vi "Create System Config Files.vi"(4 "IO's config":string="test setting", 6 "Test Setting":string="test setting", 8 "count":string="Calib", 9 "Settings":string="Settings", 10 "User Data":string="user data", 11 "file path (use dialog)":path=path "C:/Documents and Settings/Owner/Desktop") -> (3 "Path 2":T1)   [LabVIEW 2023]
uses:
  Controls/all path.ctl
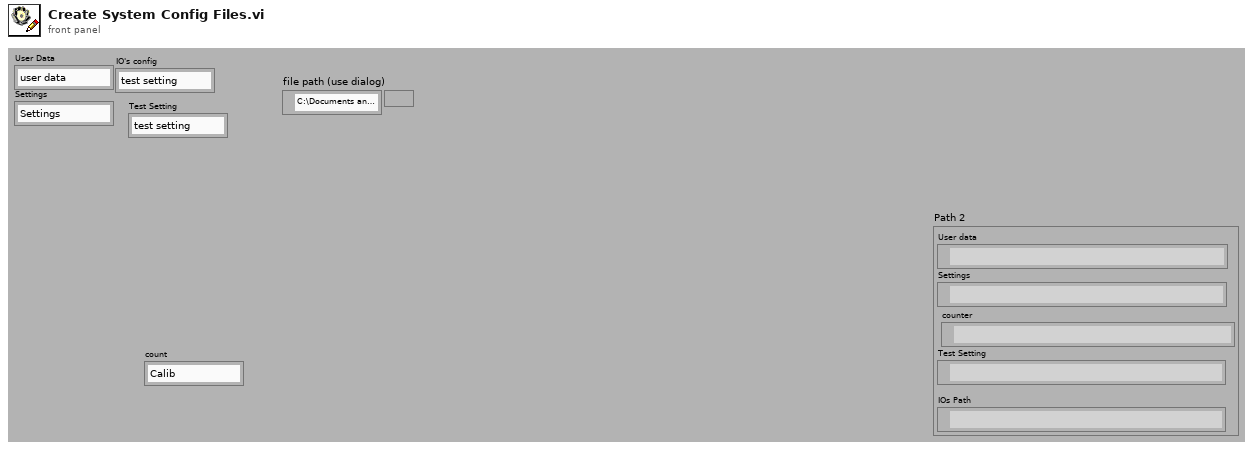
[diagram p1: front panel]
types:
  T1 = typedef "all path.ctl" = cluster{"User data":path, "Settings":path, "counter":path, "Test Setting":path, "IOs Path":path}
  T2 = enum16{"open", "replace", "create", "open or create", "replace or create", "replace or create with confirmation"}
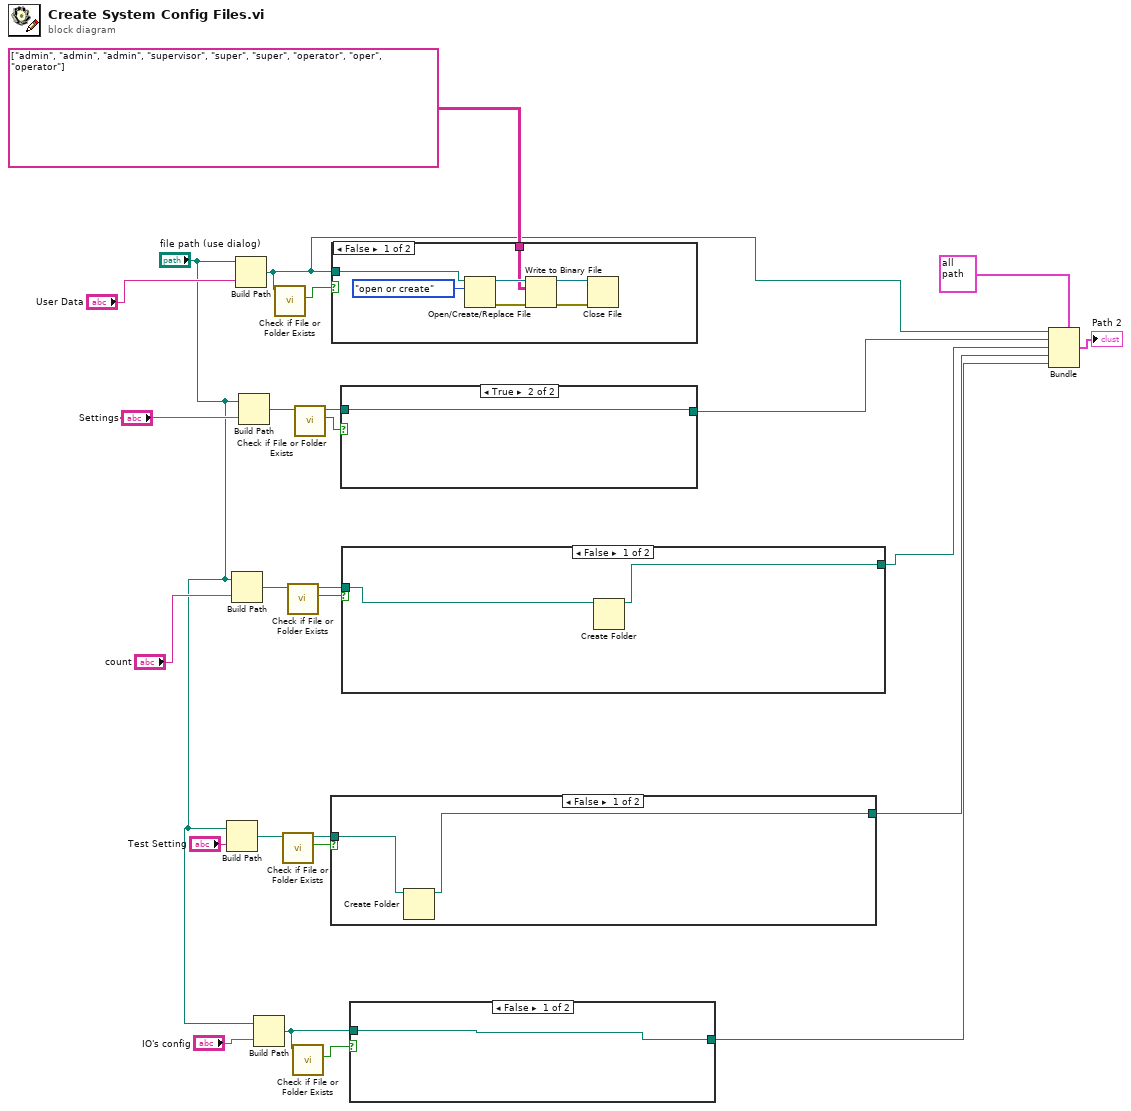
[diagram p0: block diagram]
diagram:
  n1 = Build Path(base path="file path (use dialog)", name or relative path="Test Setting") -> (appended path=w9:path)
  n2 = Build Path(base path="file path (use dialog)", name or relative path="count") -> (appended path=w18:path)
  n3 = Build Path(base path="file path (use dialog)", name or relative path="User Data") -> (appended path=w12:path)
  n4 = Build Path(base path="file path (use dialog)", name or relative path="Settings") -> (appended path=w22:path)
  n5 = Build Path(base path="file path (use dialog)", name or relative path="IO's config") -> (appended path=w2:path)
  n6 = call <vilib>:"Check if File or Folder Exists.vi"("path"=w12) -> ("file or folder exists?"=w13:bool)  [unwired: 8 in, 2 out]
  n7 = call <vilib>:"Check if File or Folder Exists.vi"("path"=w9) -> ("file or folder exists?"=w10:bool, "dup path"=w11:path)  [unwired: 8 in, 1 out]
  n8 = call <vilib>:"Check if File or Folder Exists.vi"("path"=w18) -> ("file or folder exists?"=w17:bool, "dup path"=w16:path)  [unwired: 8 in, 1 out]
  n9 = call <vilib>:"Check if File or Folder Exists.vi"("path"=w2) -> ("file or folder exists?"=w5:bool)  [unwired: 8 in, 2 out]
  n10 = call <vilib>:"Check if File or Folder Exists.vi"("path"=w22) -> ("file or folder exists?"=w21:bool, "dup path"=w20:path)  [unwired: 8 in, 1 out]
  n11 = case shown="False" w10 {
    tunnel: w11 -> [w28 w29]
    tunnel: [w27 w29] -> w7
    frame False {
      n12 = Create Folder(path (use dialog)=w28) -> (created path=w27:path)  [unwired: 2 in, 2 out]
    }
    frame True {
    }
  }
  n13 = case shown="False" w13 {
    tunnel: string[][] [["admin", "admin", "admin"], ["supervisor", "super", "super"], ["operator", "oper", "operator"]] ("Cluster") -> [w31 _]
    tunnel: w12 -> [w30 _]
    frame False {
      n14 = Open/Create/Replace File(file path (use dialog)=w30, operation (0:open)=T2."open or create") -> (refnum out=w36:refnum<file>, error out=w35:errorcluster)  [unwired: 4 in, 1 out]
      n15 = Write to Binary File(file (use dialog)=w36, data=w31, error in=w35) -> (refnum out=w33:refnum<file>, error out=w34:errorcluster)  [unwired: 4 out]
      n16 = Close File(refnum=w33, error in=w34) -> ()  [unwired: 2 out]
    }
    frame True {
    }
  }
  n17 = case shown="True" w21 {
    tunnel: w20 -> [w37 w38]
    tunnel: [w37 w38] -> w19
    frame False {
    }
    frame True {
    }
  }
  n18 = case shown="False" w17 {
    tunnel: w16 -> [w40 w41]
    tunnel: [w39 w41] -> w14
    frame False {
      n19 = Create Folder(path (use dialog)=w40) -> (created path=w39:path)  [unwired: 2 in, 2 out]
    }
    frame True {
    }
  }
  n20 = case shown="False" w5 {
    tunnel: w2 -> [w42 w43]
    tunnel: [w42 w43] -> w1
    frame False {
    }
    frame True {
    }
  }
  n21 = Bundle(cluster=T1 {"User data"=path "", "Settings"=path "", "counter"=path "", "Test Setting"=path "", "IOs Path"=path ""} ("Path 2"), "User data"=w12, "Settings"=w19, "counter"=w14, "Test Setting"=w7, "IOs Path"=w1) -> (→"Path 2":T1)
